vi "TC560-Request.vi"(8 "error in":errorcluster, 10 "Command":string, 11 "VISA Resource Name In":refnum<visa-resource-name>) -> (0 "error out":errorcluster, 2 "Respond":string, 3 "VISA Resource Name Out":refnum<visa-resource-name>)   [LabVIEW 2018]
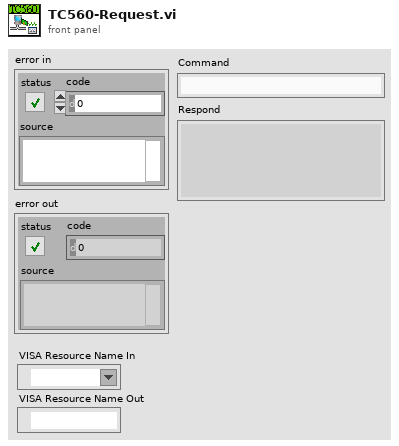
[diagram p1: front panel]
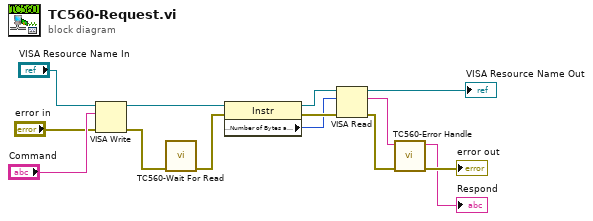
[diagram p0: block diagram]
diagram:
  n1 = VISA Write(VISA resource name="VISA Resource Name In", write buffer="Command", error in (no error)="error in") -> (VISA resource name out=w13:refnum<visa-resource-name>, error out=w14:errorcluster)  [unwired: 1 out]
  n2 = call "TC560-Wait For Read.vi"("error in"=w14) -> ("error out"=w12:errorcluster)  [unwired: 10 in]
  n3 = property class="Instr"(reference=w13, error in=w12) -> (reference out=w11:refnum<visa-resource-name>, error out=w10:errorcluster, "Serial Settings:Number of Bytes at Serial Port"=w9:u32)
  n4 = VISA Read(VISA resource name=w11, byte count=w9, error in (no error)=w10) -> (VISA resource name out=→"VISA Resource Name Out":refnum<visa-resource-name>, read buffer=w7:string, error out=w8:errorcluster)  [unwired: 1 out]
  n5 = call "TC560-Error Handle.vi"("error in"=w8, "Respond In"=w7) -> ("error out"=→"error out":errorcluster, "Respond Out"=→"Respond":string)  [unwired: 8 in]
